vi "Constants.vi"() -> ()   [LabVIEW 2015, in "Instrument Addon Shared.lvlib"]
doc: "Use this Global VI to access the GUIDs assigned to the page resources of the Custom Device."
uses:
  Instrument Addon Shared.lvlib
panel:
  in  "Tab Control":T1(tab)=enum."Data"
  in  "Array MetaData Element GUID":string="193453c7-2cce-4840-9490-648855c0cf25"
  in  "Array Data Element GUID":string="566d73be-f343-477c-b55f-6f2c19d26406"
  in  "Enable Periodic GUID":string="0766e40f-9a8b-40a8-8d2d-c67262ede28a"
  in  "Message Group GUID":string="ca2af2c4-f6de-4981-9e7c-f3a7dc921a83"
  in  "Global MetaData Channels GUID":string="6a1d81ec-ec4c-425e-ab83-1c5b7af136d6"
  in  "Message Status GUID":string="a618186b-06ee-4c96-843e-7b3da3094e99"
  in  "Serial Protocol GUID Disabled":string="02db78c0-2fa5-4cb3-bdc4-0f140d052e7d"
  in  "MetaData Channel GUID":string="1d30d097-ad35-4eb1-81b5-9d3a9f7f2d88"
  in  "Data Channel GUID":string="b473b5ce-647b-4798-814d-3247489a3409"
  in  "Response GUID":string="e90b6266-233a-4552-94b4-54222f1875a2"
  in  "Command GUID":string="9428600d-6a85-43b8-aaac-a755da7e0c9b"
  in  "Error Code GUID":string="c36593c7-9ffd-4a3f-8db5-ade8f2d84760"
  in  "Trigger GUID":string="74948967-ac25-4bb0-8b12-32de2b2e343b"
  in  "Message Channels GUID":string="72ad4790-7ba8-47a2-8882-5ec6ff5aad5f"
  in  "Message GUID":string="672eb08e-4747-4725-8ff4-4749baa5e2a0"
  in  "Serial Protocol GUID":string="5a19fd09-df16-47f0-8250-c59b5cb8c757"
  in  "CompiledSettings":string="CompiledSettings"
  in  "Global MetatData Array Name":string="Global MetaData Array"
  in  "MetaData Array Page":string="MetaData Array"
  in  "Data Array Page":string="Data Array"
  in  "TriggerChannelError":string="TriggerChannelError"
  in  "Response Not Used":string="RESPONSE NOT USED"
  in  "ProtectionSelectionError":string="ProtectionSelectionError"
  in  "WaitChannelError":string="WaitChannelError"
  in  "Enable Periodic":string="Enable Periodic"
  in  "ConfigGUID":string="ConfigGUID"
  in  "Message Group Page":string="Message Group"
  in  "Global MetatData Channel Name":string="Global MetaData"
  in  "Global MetaData Channels":string="Global MetaData Channels"
  in  "Message Status Page":string="Message Status"
  in  "MetaData Channel Page":string="MetaData"
  in  "Data Channel Page":string="Data"
  in  "Message Channels Page":string="Message Channels"
  in  "Response Page":string="Response"
  in  "Command Page":string="Command"
  in  "Error Code":string="Error Code"
  in  "Trigger Channel":string="Trigger"
  in  "Message Page":string="Message"
  in  "CmdEngineSuffix":string="_BufferedCmds"
  in  "Protocol":string="Protocol"
  in  "Decimation":string="Decimation"
  in  "Trigger.ChanPath":string="Trigger.ChanPath"
  in  "Trigger.UseChan":string="Trigger.UseChan"
  in  "VISA.Resource":string="VISA.Resource"
  in  "VISA.TermChar":string="VISA.TermChar"
  in  "VISA.Timeout":string="VISA.Timeout"
  in  "VISA.AppendTermChar":string="VISA.AppendTermChar"
  in  "VISA.EnableTermChar":string="VISA.EnableTermChar"
  in  "UDP.TargetPort":string="UDP.TargetPort"
  in  "UDP.TargetIP":string="UDP.TargetIP"
  in  "UDP.LocalPort":string="UDP.LocalPort"
  in  "UDP.LocalIP":string="UDP.LocalIP"
  in  "Data.Endian":string="Data.Endian"
  in  "Data.ExpectedString":string="Data.ExpectedString"
  in  "Data.Delimiter":string="Data.Delimiter"
  in  "Data.TypeCastType":string="Data.TypeCastType"
  in  "Data.FormatString":string="Data.FormatString"
  in  "Data.List":string="Data.List"
  in  "Data.ChanType":string="Data.ChanType"
  in  "Data.DataType":string="Data.DataType"
  in  "Msg.ProtectType":string="Msg.ProtectType"
  in  "Msg.UseProtect":string="Msg.UseProtect"
  in  "Msg.Period":string="Msg.Period"
  in  "Msg.GenType":string="Msg.GenType"
  in  "TCP.Port":string="TCP.Port"
  in  "TCP.IP":string="TCP.IP"
  in  "MetaData.Endian":string="MetaData.Endian"
  in  "MetaData.Delimiter":string="MetaData.Delimiter"
  in  "MetaData.TypeCastType":string="MetaData.TypeCastType"
  in  "MetaData.FormatString":string="MetaData.FormatString"
  in  "MetaData.List":string="MetaData.List"
  in  "MetaData.ChanType":string="MetaData.ChanType"
  in  "MetaData.DataType":string="MetaData.DataType"
  in  "Cmd.PadVal":string="Cmd.PadVal"
  in  "Cmd.PadLength":string="Cmd.PadLength"
  in  "Cmd.Pad":string="Cmd.Pad"
  in  "Cmd.LinkedGUIDs":string="Cmd.LinkedGUID"
  in  "Cmd.LinkedChans":string="Cmd.LinkedChans"
  in  "Cmd.Cmd":string="Cmd.Cmd"
  in  "Rsp.ChanPath":string="Rsp.ChanPath"
  in  "Rsp.UseChan":string="Rsp.UseChan"
  in  "Rsp.WaitType":string="Rsp.WaitType"
  in  "Rsp.WaitVal":string="Rsp.WaitVal"
  in  "Rsp.LinkedGUIDs":string="Rsp.LinkedGUIDs"
  in  "Rsp.LinkedChans":string="Rsp.LinkedChans"
  in  "Rsp.Rsp":string="Rsp.Rsp"
  in  "RS.TermChar":string="RS.TermChar"
  in  "RS.EnableWriteTermChar":string="RS.EnableWriteTermChar"
  in  "RS.EnableReadTermChar":string="RS.EnableReadTermChar"
  in  "RS.XOFF":string="RS.XOFF"
  in  "RS.XON":string="RS.XON"
  in  "RS.FlowCntrl":string="RS.FlowCntrl"
  in  "RS.StopBits":string="RS.StopBits"
  in  "RS.Parity":string="RS.Parity"
  in  "RS.DataBits":string="RS.DataBits"
  in  "RS.BaudRate":string="RS.BaudRate"
  in  "RS.Port":string="RS.Port"
  in  "Refs.MetaData":string="MetaData"
  in  "Refs.Status":string="Status"
  in  "Refs.Triggers":string="Triggers"
  in  "Refs.PeriodicEnable":string="PeriodicEnable"
  in  "Refs.Data":string="Data"
  in  "Refs.Waits":string="Waits"
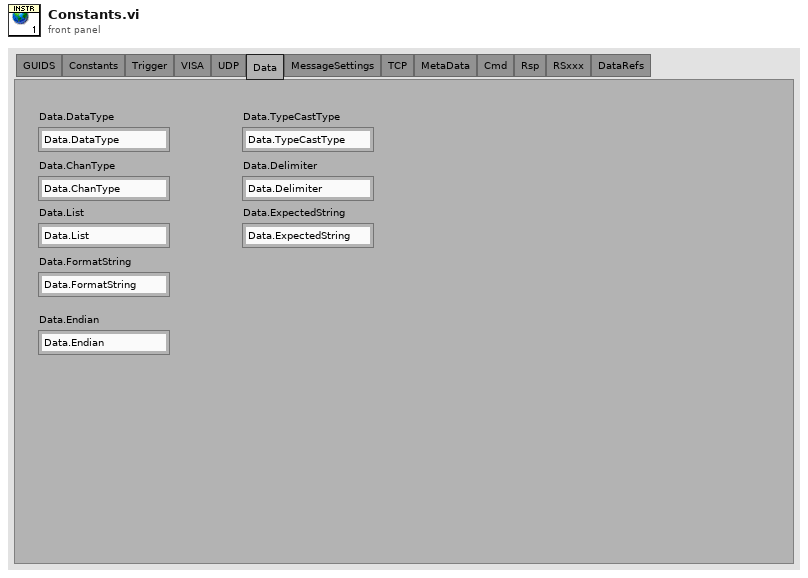
[diagram p1: front panel]
types:
  T1 = enum32{"GUIDS", "Constants", "Trigger", "VISA", "UDP", "Data", "MessageSettings", "TCP", "MetaData", "Cmd", "Rsp", "RSxxx", "DataRefs"}
diagram:
